vi "CSM - List Submodules.vi"(8 "Error In":errorcluster caption="Error in (no error)", 9 "Recursive? (T)":bool=TRUE, 11 "Parent Name":string) -> (0 "Error Out":errorcluster, 2 "Submodules":string[](array[string]), 3 "Parent Name (Dup)":string)   [LabVIEW 2017, in "Communicable State Machine.lvlib"]
doc: "Lists all submodules of the current group or module. When <b>Recursive? (T)</b> is TRUE, This VI recursively lists submodules at all levels. Otherwise, this VI only lists the direct next-level submodules.\n\n Example: The system contains the following five modules: Level1.Level2A, Level1.Level2A.Node1, Level1.Level2A.Node2, Level1.Level2B.Node1, Level1.Level2B.Node2.\n - When <b>Parent Name</b> is \"Level1\":\n If <b>Recursive? (T)</b> is True, this VI recursively lists submodules at all levels, including Level1.Level2A, Level1.Level2A.Node1, Level1.Level2A.Node2, Level1.Level2B.Node1, Level1.Level2B.Node2.\n If <b>Recursive? (T)</b> is False, this VI only lists direct next-level submodules, which only includes Level1.Level2A. Note that Level1.Level2B is not a module instance, so it is not included in the results.\n\n> [!NOTE]\n> Submodules are only valid for normal CSM modules and are invalid for modules in Worker Mode or Chain of Responsibility Mode.\n\n\n> [!NOTE] <b>CSM Submodule</b>\n>\n> There are no strict submodules in CSM. The `.` in the module name is only used to mark the logical relationship between different modules. From an actual execution perspective, each module is independent and has no hierarchical relationship. For example, modules `ModuleA` and `ModuleA.SubmoduleB` are two different modules. From the code logic perspective, they are completely independent and do not interfere with each other. However, the CSM - List Submodules VI can be used to retrieve all logical submodules of `ModuleA`, including `ModuleA.SubmoduleB`.\n>\n> It is important to note that `ModuleA` does not have to actually exist. It can serve merely as a logical group. For example, modules `Group.SubModuleA` and `Group.SubModuleB` are two different modules. From the code logic perspective, they are completely independent and do not interfere with each other. However, the CSM - List Submodules VI can be used to retrieve all logical submodules of `Group`, including `Group.SubModuleA` and `Group.SubModuleB`.\n>\n> CSM module names in Worker Mode and Chain of Responsibility Mode can also contain `.`, as this is only logical grouping and does not affect module operation.\n\n\n-- <b>Controls</b> --\n- <b>Parent Name</b>: Group or parent node name.\n- <b>Recursive? (T)</b>: Whether to recursively list submodules at all levels. The default is TRUE.\n\n-- <b>Indicators</b> --\n- <b>Parent Name (Dup)</b>: A copy of the input group or parent node name.\n- <b>Submodules</b>: List of submodule names."
uses:
  Communicable State Machine.lvlib
  _Support/CSMQ/_CSMOFGVOPER.ctl
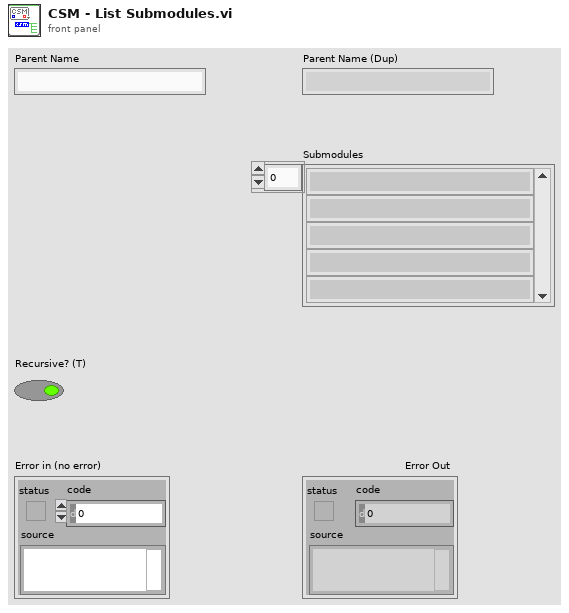
[diagram p1: front panel]
types:
  T1 = typedef "Communicable State Machine.lvlib/_CSMOFGVOPER.ctl" = enum16{"Create If not Exist", "Get By Name", "List", "Check If Name Exists", "Release", "Module Status", "Create Status Event Handler", "Destroy Status Event Handler", "Clear Invalid Objs"}
  T2 = typedef "Communicable State Machine.lvlib/_CSMObj.ctl" = cluster{"info":T3, "Refs":T5}
  T3 = typedef "Communicable State Machine.lvlib/_CSMObj-Info.ctl" = cluster{"Module Name":string, "Requested Name":string, "Group Name":string, "Mode":T4, "Allowed Messages":string[]}
  T4 = typedef "Communicable State Machine.lvlib/_CSM_MODE.ctl" = enum16{"Not Exist", "Stand Alone", "CSM", "Worker", "Worker Agent", "Chain Node", "Chain"}
  T5 = typedef "Communicable State Machine.lvlib/_CSMObj-Refs.ctl" = cluster{"WatchDogQ":refnum<queue>, "CSMDataDVR":refnum<data-value>, "Queue":T6, "GroupDataDVR":refnum<data-value>, "TagMap":refnum<data-value>, "ExitEvent":refnum<user-event>, "NewStateEvent":refnum<user-event>, "StatusEvent":refnum<user-event>, "InterruptEvent":refnum<user-event>}
  T6 = typedef "Communicable State Machine.lvlib/Priority Queue.ctl" = cluster{"HPriorityQ":refnum<queue>, "LowPriorityQ":refnum<queue>}
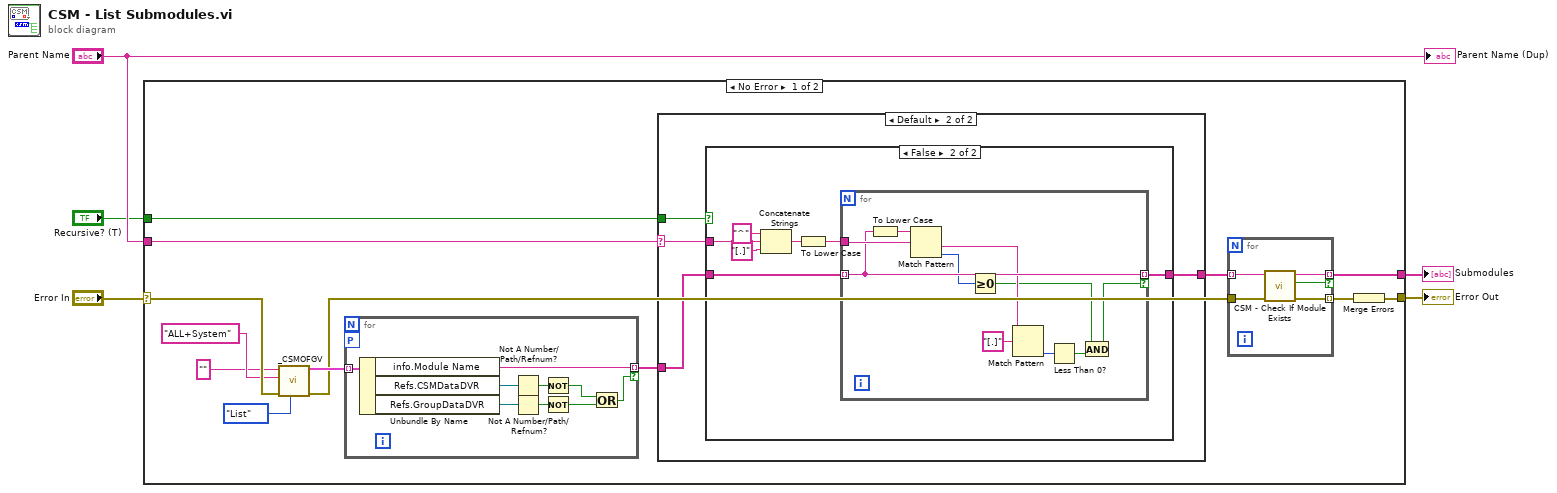
[diagram p0: block diagram]
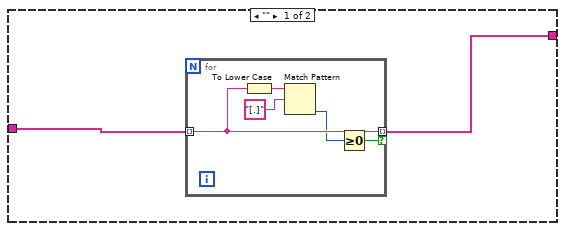
[diagram p2: hidden frame]
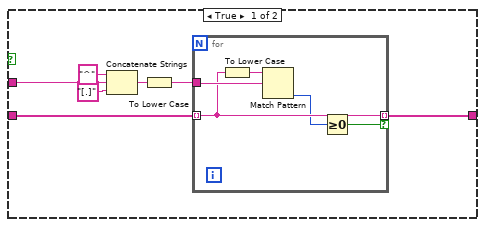
[diagram p3: hidden frame]
diagram:
  n1 = case shown="No Error" "Error In" {
    selector: "Error In" -> [w17 w73]
    tunnel: [w7 w73] -> w4
    tunnel: "Parent Name" -> [w18 _]
    tunnel: [w11 _] -> w2
    tunnel: "Recursive? (T)" -> [w6 _]
    frame No Error {
      n2 = call "_CSMOFGV.vi"("Operation"=_CSMOFGVOPER."List", "Error In"=w17, "Reference"="ALL+System", "Name (\"\" to Use UUID) In"="" ("Name(\"\" to use uuid) in")) -> ("error out"=w8:errorcluster, "Array"=w16:T2[])  [unwired: 5 in, 1 out]
      n3 = for {
        tunnel: w16 -> [w27] mode=indexing
        tunnel: [w26] -> w12 mode=indexing if=w24
        workers-P: _ -> [_]
        n4 = Unbundle By Name(w27) -> ("info.Module Name"=w26:string, "Refs.CSMDataDVR"=w21:refnum<data-value>, "Refs.GroupDataDVR"=w20:refnum<data-value>)
        n5 = Not A Number/Path/Refnum?(number/path/refnum=w21) -> (NaN/Path/Refnum?=w25:bool)
        n6 = Not A Number/Path/Refnum?(number/path/refnum=w20) -> (NaN/Path/Refnum?=w22:bool)
        n7 = Not(x=w25) -> (.not. x?=w23:bool)
        n8 = Not(x=w22) -> (.not. x?=w19:bool)
        n9 = Or(x=w23, y=w19) -> (x .or. y?=w24:bool)
      }
      n10 = case shown="Default" w18 {
        selector: w18 -> [_ w43]
        tunnel: [w34 w42] -> w10
        tunnel: w12 -> [w33 w41]
        tunnel: w6 -> [_ w40]
        frame "" {
          n11 = for {
            tunnel: w33 -> [w39] mode=indexing
            tunnel: [w39] -> w34 mode=indexing if=w36
            n12 = To Lower Case(string=w39) -> (all lower case string=w38:string)
            n13 = Match Pattern(string=w38, regular expression="[.]" ("string")) -> (offset past match=w37:i32)  [unwired: 1 in, 3 out]
            n14 = Greater Or Equal To 0?(x=w37) -> (x >= 0?=w36:bool)
          }
        }
        frame Default {
          n15 = case shown="False" w40 {
            tunnel: w43 -> [w50 w62]
            tunnel: [w49 w61] -> w42
            tunnel: w41 -> [w44 w56]
            frame True {
              n16 = Concatenate Strings("^" ("string"), w50, "[.]" ("string")) -> (w48:string)
              n17 = To Lower Case(string=w48) -> (all lower case string=w45:string)
              n18 = for {
                tunnel: w45 -> [w55]
                tunnel: w44 -> [w54] mode=indexing
                tunnel: [w54] -> w49 mode=indexing if=w51
                n19 = To Lower Case(string=w54) -> (all lower case string=w53:string)
                n20 = Match Pattern(string=w53, regular expression=w55) -> (offset past match=w52:i32)  [unwired: 1 in, 3 out]
                n21 = Greater Or Equal To 0?(x=w52) -> (x >= 0?=w51:bool)
              }
            }
            frame False {
              n22 = Concatenate Strings("^" ("string"), w62, "[.]" ("string")) -> (w60:string)
              n23 = To Lower Case(string=w60) -> (all lower case string=w57:string)
              n24 = for {
                tunnel: w57 -> [w72]
                tunnel: w56 -> [w71] mode=indexing
                tunnel: [w71] -> w61 mode=indexing if=w66
                n25 = To Lower Case(string=w71) -> (all lower case string=w70:string)
                n26 = Match Pattern(string=w70, regular expression=w72) -> (after substring=w68:string, offset past match=w69:i32)  [unwired: 1 in, 2 out]
                n27 = Greater Or Equal To 0?(x=w69) -> (x >= 0?=w65:bool)
                n28 = Match Pattern(string=w68, regular expression="[.]") -> (offset past match=w64:i32)  [unwired: 1 in, 3 out]
                n29 = Less Than 0?(x=w64) -> (x < 0?=w63:bool)
                n30 = And(x=w65, y=w63) -> (x .and. y?=w66:bool)
              }
            }
          }
        }
      }
      n31 = for {
        tunnel: [w31] -> w11 mode=indexing if=w30
        tunnel: w10 -> [w32] mode=indexing
        tunnel: [w29] -> w9 mode=indexing
        tunnel: w8 -> [w28]
        n32 = call "CSM - Check If Module Exists.vi"("Error In"=w28, "CSM Name"=w32) -> ("error out"=w29:errorcluster, "Exist?"=w30:bool, "CSM Name (Dup)"=w31:string)  [unwired: 7 in]
      }
      n33 = Merge Errors(w9) -> (w7:errorcluster)
    }
    frame Error {
    }
  }
  "Error Out" <- w4
  "Submodules" <- w2
  "Parent Name (Dup)" <- "Parent Name"
